vi "AUTO_Encoder_In_Range_Check.vi"(9 "Right Encoder":i32, 10 "Left Encoder":i32, 11 "PostionTarget(Counts)":i32) -> (3 "Boolean":bool)   [LabVIEW 2017, in "Autonomous.lvlib"]
uses:
  Autonomous.lvlib
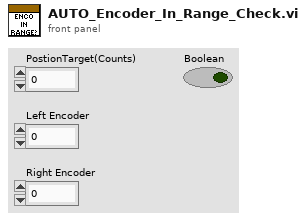
[diagram p1: front panel]
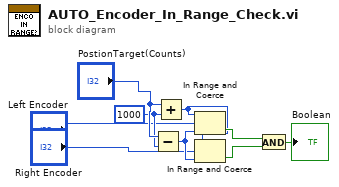
[diagram p0: block diagram]
diagram:
  w4 = 1000 ("y")
  n1 = Subtract(x="PostionTarget(Counts)", y=w4) -> (x-y=w7:i32)
  n2 = Add(x="PostionTarget(Counts)", y=w4) -> (x+y=w6:i32)
  n3 = In Range and Coerce(upper limit=w6, x="Left Encoder", lower limit=w7) -> (In Range?=w9:bool)  [unwired: 1 out]
  n4 = In Range and Coerce(upper limit=w6, x="Right Encoder", lower limit=w7) -> (In Range?=w8:bool)  [unwired: 1 out]
  n5 = And(x=w9, y=w8) -> (x .and. y?=→"Boolean":bool)
